vi "Create Collection.vi"(4 "Interactive (T)":bool=TRUE, 5 "Test Runner.Collection in":refnum<class "Test Runner.Collection.lvclass">, 6 "Verbose (F)":bool, 7 "Test Report":refnum<class "Test Report.lvclass">, 8 "error in (no error)":errorcluster, 9 "Test Runners":refnum<class "Test Runner.lvclass">[](array[class]), 10 "Test Runner 2":refnum<class "Test Runner.lvclass">, 11 "Test Runner 1":refnum<class "Test Runner.lvclass">) -> (0 "error out":errorcluster, 3 "Test Runner.Collection out":refnum<class "Test Runner.Collection.lvclass">)   [LabVIEW 2013, in "Caraya.lvlib" / "Test Runner.Collection.lvclass"]
uses:
  Test Runner.Collection.lvclass
  Test Runner/Test Runner.lvclass
  Test Report/Test Report.lvclass
  Test Runner/Test Runner.lvclass/Test Runner.ctl
  Test Runner.Collection.lvclass/Test Runner.Collection.ctl
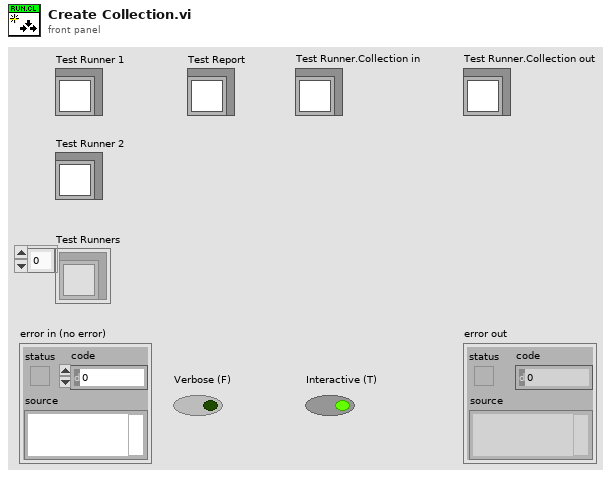
[diagram p1: front panel]
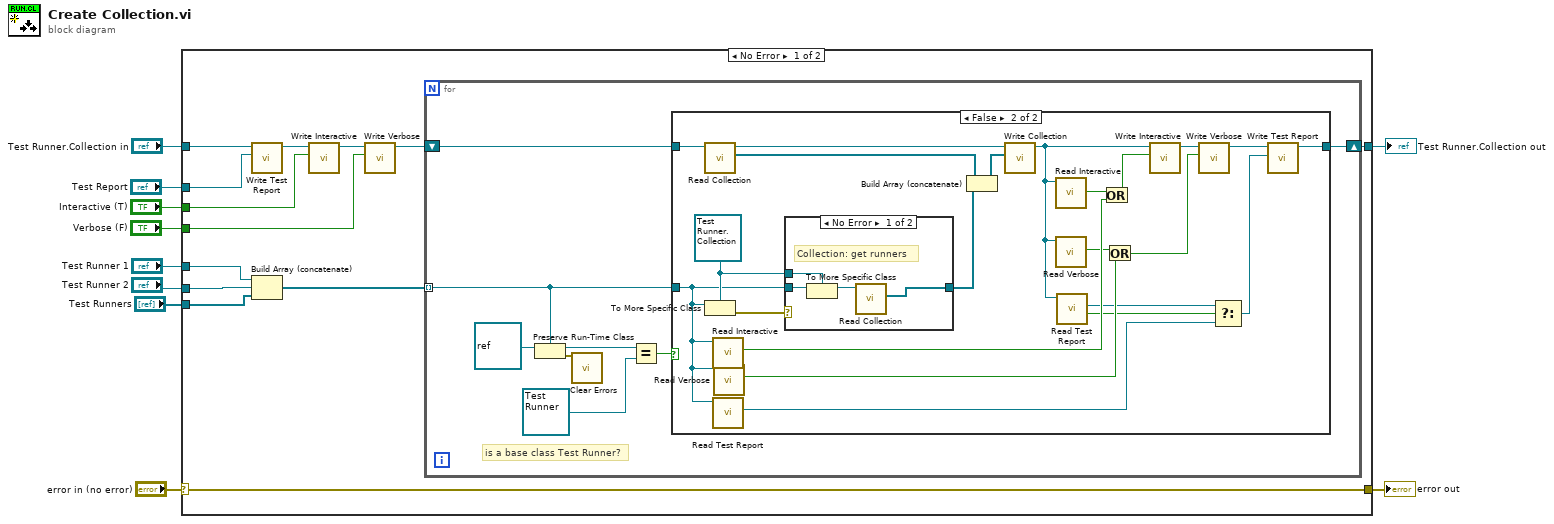
[diagram p0: block diagram]
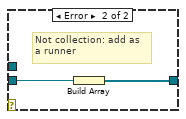
[diagram p3: hidden frame]
diagram:
  n1 = case shown="No Error" "error in (no error)" {
    selector: "error in (no error)" -> [w11 w62]
    tunnel: [w23 w61] -> w10
    tunnel: "Test Runner 2" -> [w22 _]
    tunnel: "Test Runner 1" -> [w20 _]
    tunnel: "Test Runners" -> [w19 _]
    tunnel: "Test Runner.Collection in" -> [w18 w61]
    tunnel: "Test Report" -> [w17 _]
    tunnel: "Interactive (T)" -> [w16 _]
    tunnel: "Verbose (F)" -> [w12 _]
    tunnel: [w11 w62] -> w1
    frame No Error {
      n2 = call "Write Test Report.vi"("Test Report"=w17, "Test Runner in"=w18) -> ("Test Runner out"=w14:refnum<class "Test Runner.Collection.lvclass">)  [unwired: 9 in]
      n3 = Build Array (concatenate)(w20, w22, w19) -> (w21:refnum<class "Test Runner.lvclass">[])
      n4 = call "Write Interactive.vi"("Interactive"=w16, "Test Runner in"=w14) -> ("Test Runner out"=w15:refnum<class "Test Runner.Collection.lvclass">)  [unwired: 9 in]
      n5 = call "Write Verbose.vi"("Verbose"=w12, "Test Runner in"=w15) -> ("Test Runner out"=w13:refnum<class "Test Runner.Collection.lvclass">)  [unwired: 9 in]
      n6 = for {
        tunnel: w21 -> [w25] mode=indexing
        shift-right: [w31] -> w23
        shift-left: w13 -> [w24]
        # "is a base class Test Runner?"
        n7 = Preserve Run-Time Class(object in=refnum<class> refnum ("LabVIEW Object"), 2:w25) -> (object out=w29:refnum<class "Test Runner.lvclass">, error out=w26:errorcluster)  [unwired: 1 in]
        n8 = call <vilib>:"Clear Errors.vi"("error in (no error)"=w26) -> ()  [unwired: 6 in, 1 out]
        n9 = Equal?(x=w29, y=refnum<class "Test Runner.lvclass"> refnum ("Caraya.lvlib:Test Runner.lvclass")) -> (x = y?=w27:bool)
        n10 = case shown="False" w27 {
          tunnel: [w32 w38] -> w31
          tunnel: w24 -> [w32 w48]
          tunnel: w25 -> [_ w40]
          frame True {
          }
          frame False {
            w52 = refnum<class "Test Runner.Collection.lvclass"> refnum ("Collection")
            n11 = call "Read Collection.vi"("Test Runner.Collection in"=w48) -> ("Test Runners"=w50:refnum<class "Test Runner.lvclass">[], "Test Runner.Collection out"=w49:refnum<class "Test Runner.Collection.lvclass">)  [unwired: 9 in]
            n12 = To More Specific Class(target class=w52, reference=w40) -> (error out=w51:errorcluster)  [unwired: 1 in, 1 out]
            n13 = call "Read Interactive.vi"("Test Runner in"=w40) -> ("Interactive"=w45:bool)  [unwired: 9 in, 1 out]
            n14 = call "Read Test Report.vi"("Test Runner in"=w40) -> ("Test Report"=w34:refnum<class "Test Report.lvclass">)  [unwired: 8 in, 2 out]
            n15 = call "Read Verbose.vi"("Test Runner in"=w40) -> ("Verbose"=w42:bool)  [unwired: 9 in, 1 out]
            n16 = case shown="No Error" w51 {
              tunnel: w40 -> [w57 w59]
              tunnel: [w58 w60] -> w53
              tunnel: w52 -> [w56 _]
              frame No Error {
                # "Collection: get runners"
                n17 = To More Specific Class(target class=w56, reference=w57) -> (specific class reference=w55:refnum<class "Test Runner.Collection.lvclass">)  [unwired: 1 in, 1 out]
                n18 = call "Read Collection.vi"("Test Runner.Collection in"=w55) -> ("Test Runners"=w58:refnum<class "Test Runner.lvclass">[])  [unwired: 9 in, 1 out]
              }
              frame Error {
                # "Not collection: add as\na runner"
                n19 = Build Array(w59) -> (w60:refnum<class "Test Runner.lvclass">[])
              }
            }
            n20 = Build Array (concatenate)(w50, w53) -> (w54:refnum<class "Test Runner.lvclass">[])
            n21 = call "Write Collection.vi"("Collection"=w54, "Test Runner.Collection in"=w49) -> ("Test Runner.Collection out"=w37:refnum<class "Test Runner.Collection.lvclass">)  [unwired: 8 in, 1 out]
            n22 = call "Read Interactive.vi"("Test Runner in"=w37) -> ("Interactive"=w47:bool)  [unwired: 9 in, 1 out]
            n23 = call "Read Verbose.vi"("Test Runner in"=w37) -> ("Verbose"=w43:bool)  [unwired: 9 in, 1 out]
            n24 = call "Read Test Report.vi"("Test Runner in"=w37) -> ("defined"=w36:bool, "Test Report"=w35:refnum<class "Test Report.lvclass">)  [unwired: 8 in, 1 out]
            n25 = Or(x=w47, y=w45) -> (x .or. y?=w46:bool)
            n26 = Or(x=w43, y=w42) -> (x .or. y?=w41:bool)
            n27 = call "Write Interactive.vi"("Interactive"=w46, "Test Runner in"=w37) -> ("Test Runner out"=w44:refnum<class "Test Runner.Collection.lvclass">)  [unwired: 9 in]
            n28 = call "Write Verbose.vi"("Verbose"=w41, "Test Runner in"=w44) -> ("Test Runner out"=w39:refnum<class "Test Runner.Collection.lvclass">)  [unwired: 9 in]
            n29 = Select(t=w35, s=w36, f=w34) -> (s? t:f=w33:refnum<class "Test Report.lvclass">)
            n30 = call "Write Test Report.vi"("Test Report"=w33, "Test Runner in"=w39) -> ("Test Runner out"=w38:refnum<class "Test Runner.Collection.lvclass">)  [unwired: 9 in]
          }
        }
      }
    }
    frame Error {
    }
  }
  "Test Runner.Collection out" <- w10
  "error out" <- w1
